vi "Read Config VI.vi"(8 "error in (no error)":errorcluster, 11 "ProjectLoader in":refnum<class "ProjectLoader.lvclass">) -> (0 "error out":errorcluster, 2 "VI Refnum":refnum<vi>, 3 "ProjectLoader out":refnum<class "ProjectLoader.lvclass">)   [LabVIEW 2015, in "ProjectLoader.lvclass"]
uses:
  ProjectLoader.lvclass
  Config VI.vi
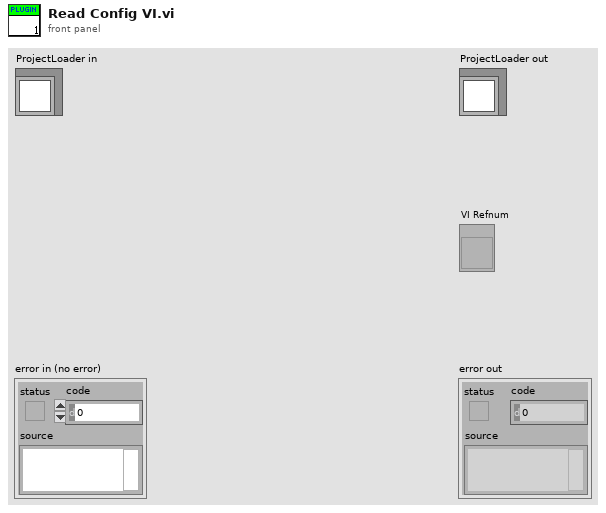
[diagram p1: front panel]
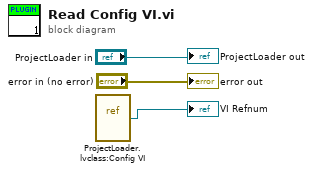
[diagram p0: block diagram]
diagram:
  n1 = vi-ref "ProjectLoader.lvclass:Config VI.vi"() -> (→"VI Refnum":refnum<vi>)
  "error out" <- "error in (no error)"
  "ProjectLoader out" <- "ProjectLoader in"
